vi "Variant Value to dot Net.vi"(7 "image path":path, 8 "error in (no error)":errorcluster, 10 "element":variant, 11 "GridColumn in":refnum<class "GridColumn.lvclass">) -> (0 "error out":errorcluster, 3 ".NET object":refnum<k24>)   [LabVIEW 2013, in "DataGrid.lvlib" / "DataTable.lvclass"]
uses:
  DataTable.lvclass
  GridColumn/GridColumn.lvclass
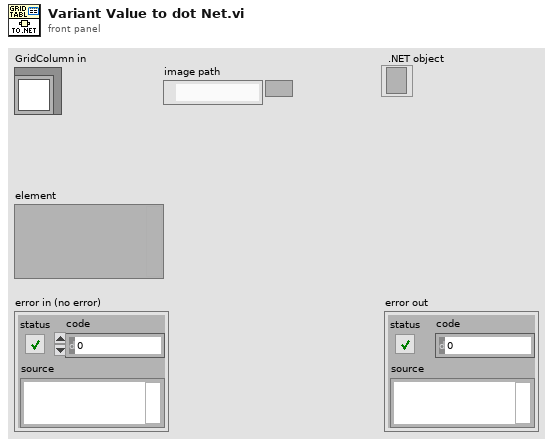
[diagram p1: front panel]
types:
  T1 = typedef "DataGrid.lvlib/GridColumn.lvclass/ColumnType.ctl" = enum16{"string", "image", "check", "numeric", "timestamp", "button", "combo", "link"}
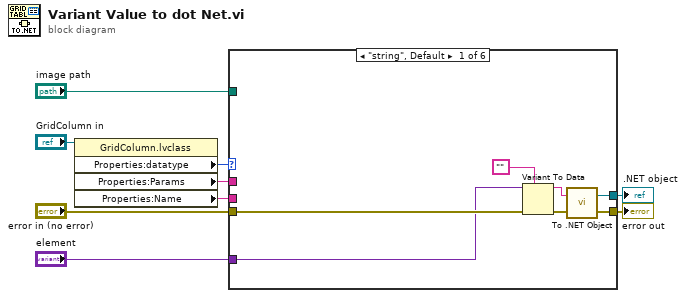
[diagram p0: block diagram]
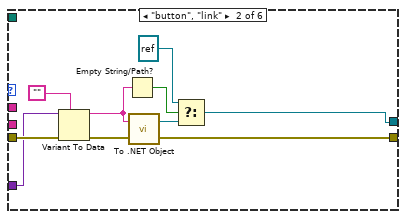
[diagram p2: hidden frame]
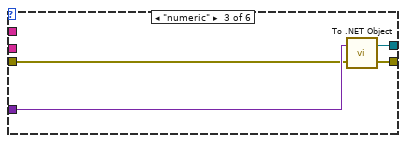
[diagram p3: hidden frame]
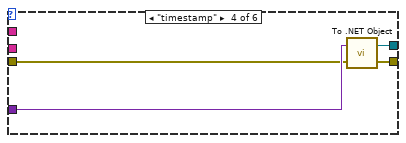
[diagram p4: hidden frame]
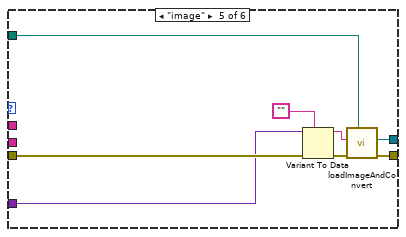
[diagram p5: hidden frame]
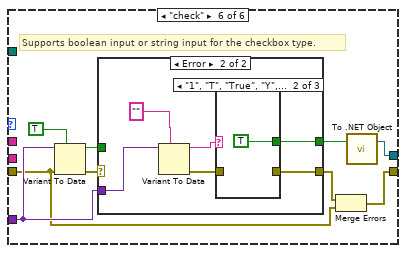
[diagram p6: hidden frame]
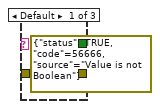
[diagram p8: hidden frame]
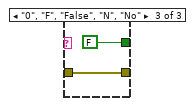
[diagram p9: hidden frame]
diagram:
  n1 = property class="GridColumn.lvclass"(reference="GridColumn in") -> ("Properties:datatype"=w6:T1, "Properties:Params"=w7:string, "Properties:Name"=w8:string)  [unwired: 1 in, 2 out]
  n2 = case shown="\"string\", Default" w6 {
    tunnel: "element" -> [w13 w23 w28 w32 w38 w46]
    tunnel: [w12 w20 w29 w33 w42 w51] -> w2
    tunnel: "error in (no error)" -> [w16 w26 w27 w31 w40 w44]
    tunnel: [w14 w24 w30 w34 w41 w43] -> w4
    tunnel: w7 -> [_ _ _ _ _ _]
    tunnel: w8 -> [_ _ _ _ _ _]
    tunnel: "image path" -> [_ _ _ _ w35 _]
    frame "string", Default {
      n3 = Variant To Data(error in=w16, type="", Variant=w13) -> (data=w11:string, error out=w15:errorcluster)
      n4 = call <vilib>:"To .NET Object.vi"("error in (no error)"=w15, "anything"=w11) -> ("error out"=w14:errorcluster, ".NET object"=w12:refnum<k24>)
    }
    frame "button", "link" {
      n5 = Variant To Data(error in=w26, type="", Variant=w23) -> (data=w17:string, error out=w25:errorcluster)
      n6 = Empty String/Path?(string/path=w17) -> (empty?=w22:bool)
      n7 = call <vilib>:"To .NET Object.vi"("error in (no error)"=w25, "anything"=w17) -> ("error out"=w24:errorcluster, ".NET object"=w21:refnum<k24>)
      n8 = Select(t=refnum<k24> refnum, s=w22, f=w21) -> (s? t:f=w20:refnum<k24>)
    }
    frame "numeric" {
      n9 = call <vilib>:"To .NET Object.vi"("error in (no error)"=w27, "anything"=w28) -> ("error out"=w30:errorcluster, ".NET object"=w29:refnum<k24>)
    }
    frame "timestamp" {
      n10 = call <vilib>:"To .NET Object.vi"("error in (no error)"=w31, "anything"=w32) -> ("error out"=w34:errorcluster, ".NET object"=w33:refnum<k24>)
    }
    frame "image" {
      n11 = Variant To Data(error in=w40, type="", Variant=w38) -> (data=w36:string, error out=w39:errorcluster)
      n12 = call "loadImageAndConvert.vi"("image path"=w35, "error in (no error)"=w39, "name or relative path"=w36) -> ("error out"=w41:errorcluster, ".NET object"=w42:refnum<k24>)  [unwired: 7 in]
    }
    frame "check" {
      # "Supports boolean input or string input for the checkbox type."
      n13 = Variant To Data(error in=w44, type=TRUE, Variant=w46) -> (data=w47:bool, error out=w48:errorcluster)
      n14 = case shown="Error" w48 {
        selector: w48 -> [w53 _]
        tunnel: [w52 w59] -> w50
        tunnel: [w53 w54] -> w45
        tunnel: w47 -> [w52 _]
        tunnel: w46 -> [_ w57]
        frame No Error {
        }
        frame Error {
          n15 = Variant To Data(type="", Variant=w57) -> (data=w58:string, error out=w55:errorcluster)  [unwired: 1 in]
          n16 = case shown="\"1\", \"T\", \"True\", \"Y\", \"Yes\"" w58 {
            tunnel: [_ TRUE FALSE] -> w59
            tunnel: w55 -> [_ _ w62]
            tunnel: [errorcluster {"status"=TRUE, "code"=56666, "source"="Value is not Boolean"} ("error out") _ w62] -> w54
            frame Default {
            }
            frame "1", "T", "True", "Y", "Yes" {
            }
            frame "0", "F", "False", "N", "No" {
            }
          }
        }
      }
      n17 = Merge Errors(w45, w44) -> (w43:errorcluster)
      n18 = call <vilib>:"To .NET Object.vi"("anything"=w50) -> (".NET object"=w51:refnum<k24>)  [unwired: 1 in, 1 out]
    }
  }
  "error out" <- w4
  ".NET object" <- w2
